vi "2d angular offset radians.vi"(8 "Vector 2":dbl[](array[numeric]), 11 "Vector 1":dbl[](array[numeric])) -> (2 "Offset Angle":dbl)   [LabVIEW 2011]
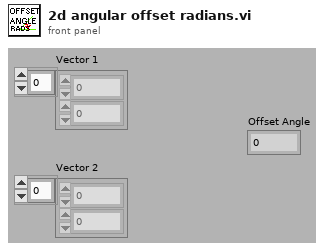
[diagram p1: front panel]
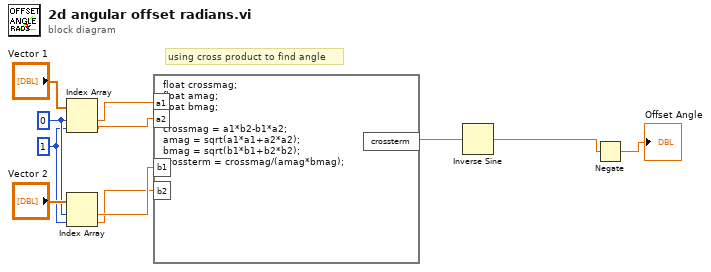
[diagram p0: block diagram]
diagram:
  w8 = 1 ("index")
  w9 = 0 ("index")
  # "using cross product to find angle"
  n1 = Index Array(array="Vector 1", index #1=w9, index #2=w8) -> (element #1=w7:dbl, element #2=w6:dbl)
  n2 = Index Array(array="Vector 2", index #1=w9, index #2=w8) -> (element #1=w5:dbl, element #2=w4:dbl)
  n3 = formula code="float crossmag;\nfloat amag;\nfloat bmag;\n\ncrossmag = a1*b2-b1*a2;\namag = sqrt(a1*a1+a2*a2);\nbmag = sqrt(b1*b1+b2*b2);\ncrossterm = crossmag/(amag*bmag);"("a1"=w7, "a2"=w6, "b1"=w5, "b2"=w4) -> ("crossterm"=w3:dbl)
  n4 = Inverse Sine(1:w3) -> (0:w1:dbl)
  n5 = Negate(x=w1) -> (-x=→"Offset Angle":dbl)
